vi "main.vi"() -> ()   [LabVIEW 2020]
uses:
  midi-ui/midi-ui.lvclass
  <vilib>/addons/_JKI Toolkits/State Machine/_JKI_lib_State_Machine.llb/Select State(s)_err__jki_lib_state_machine.vi
  midi-file/midi-file.lvclass
  midi/midi.lvclass
  midiPlayer/midiPlayer.lvclass
  midi-file-events/midi-file-events.lvclass
panel:
  out "File Name":string
  in  "Connect":bool
  in  "Midi Device":u32 caption="Numeric"
  in  "File Open":bool
  in  "Stop":bool
  in  "Pause":bool
  in  "Play":bool
  out "Connected?":bool
  in  "Exit":bool
  out "picture":picture
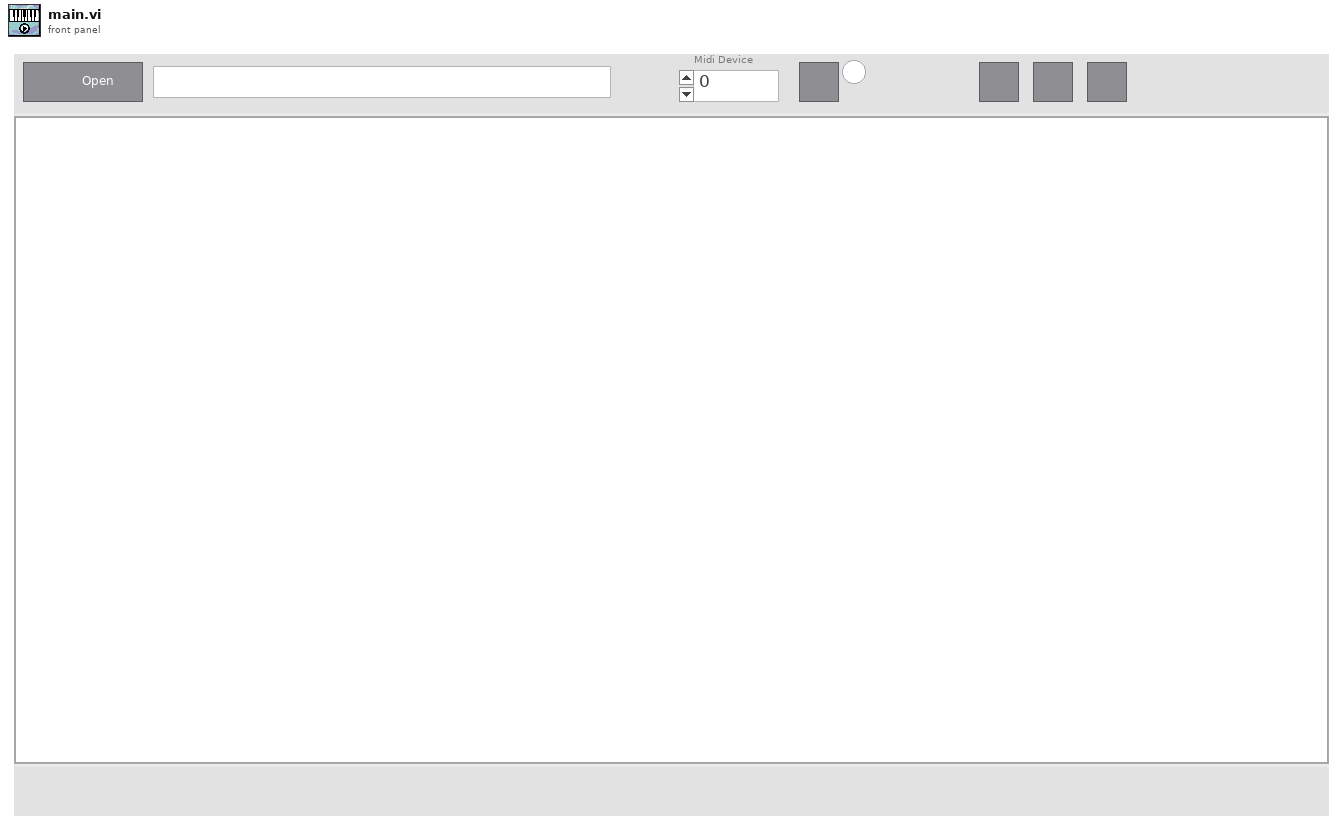
[diagram p1: front panel]
types:
  T1 = enum32{"Invalid", "Standard", "Closed", "Hidden", "Minimized", "Maximized"}
  T2 = enum32{"invalid app kind", "Development System", "Run Time System", "Student Edition", "Embedded LabVIEW", "Evaluation", "Custom"}
  T3 = cluster{"Core":cluster{"Current VI Reference":refnum<vi>, "Close Panel on Exit?":bool}, "MIDI UI":refnum<class "midi-ui.lvclass">, "midi-file-events":refnum<class "midi-file-events.lvclass">, "MIDI FILE":refnum<class "midi-file.lvclass">, "MIDI":refnum<class "midi.lvclass">, "midi connected?":bool, "midiPlayer":refnum<class "midiPlayer.lvclass">}
  T4 = cluster{"Current VI Reference":refnum<vi>, "Close Panel on Exit?":bool}
  T5 = typedef "configuration.ctl" = cluster{"Position":enum16{"Top", "Left", "Botom", "Right"}, "Note Length":dbl}
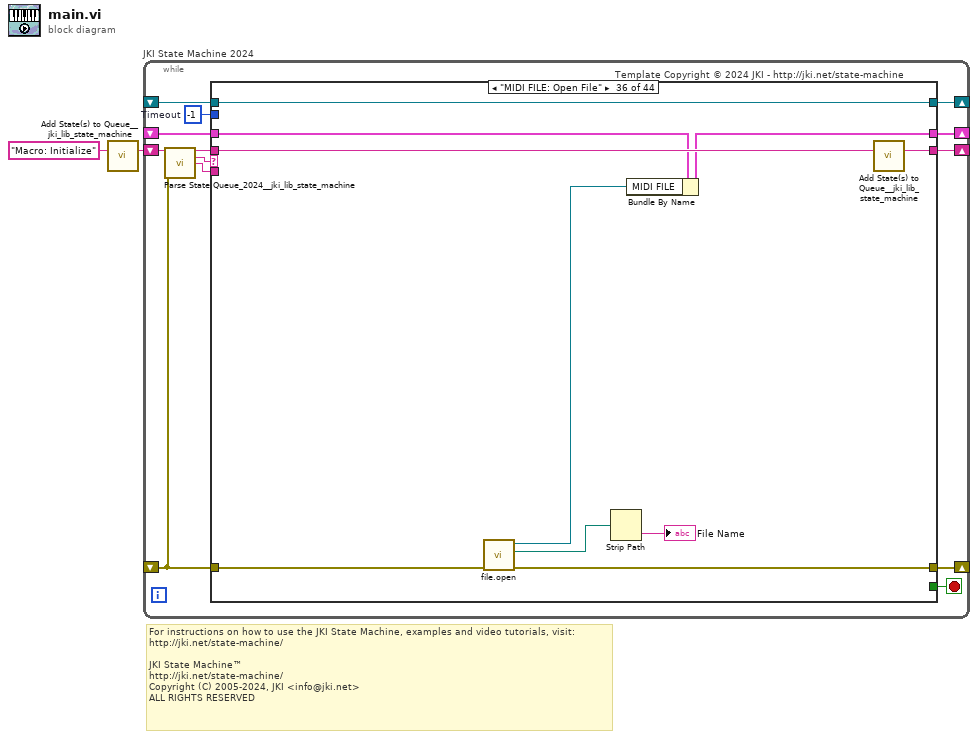
[diagram p0: block diagram]
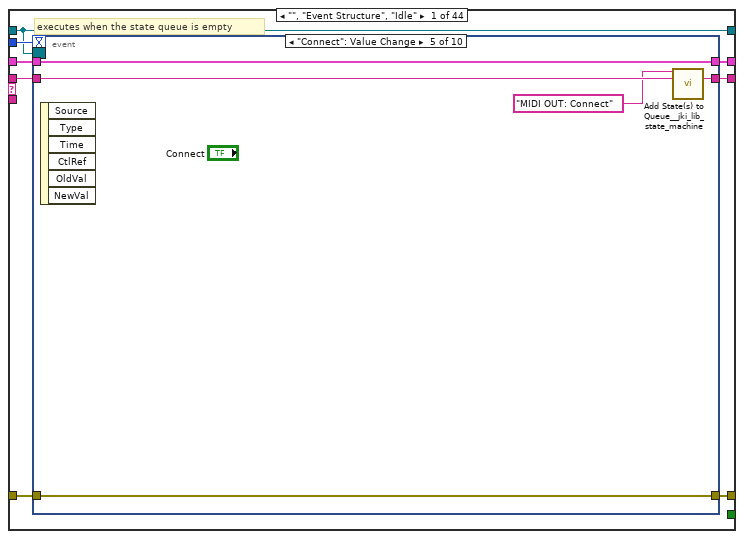
[diagram p2: hidden frame]
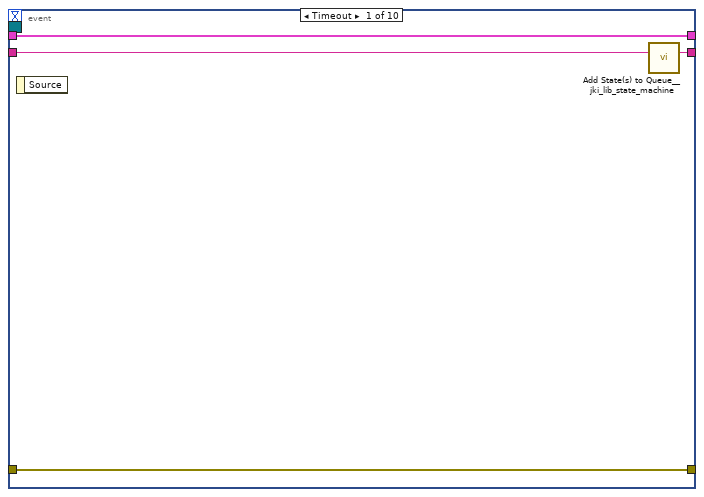
[diagram p3: hidden frame]
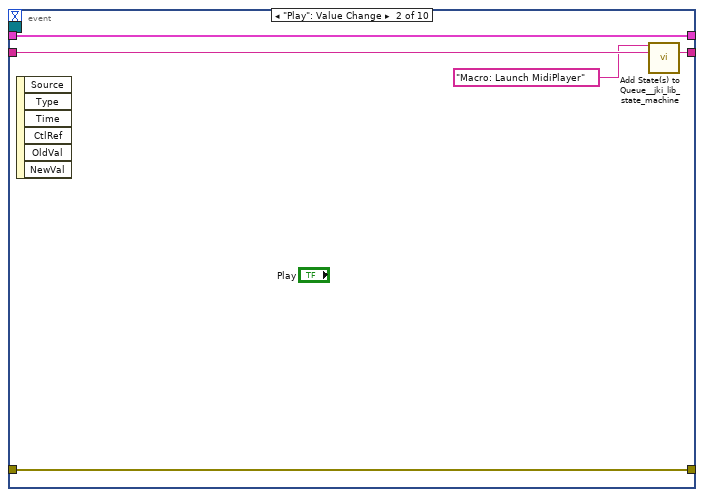
[diagram p4: hidden frame]
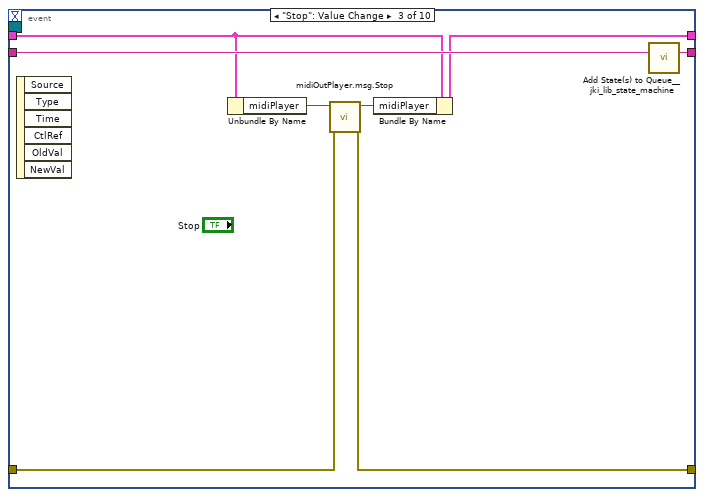
[diagram p5: hidden frame]
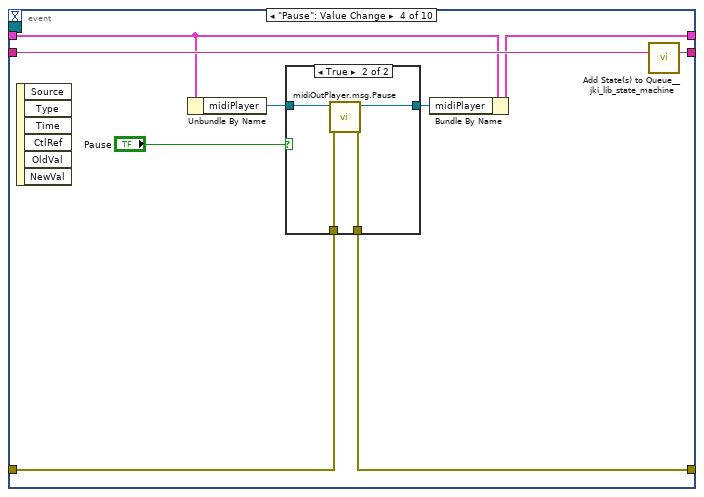
[diagram p6: hidden frame]
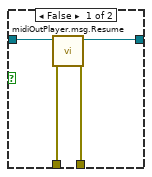
[diagram p7: hidden frame]
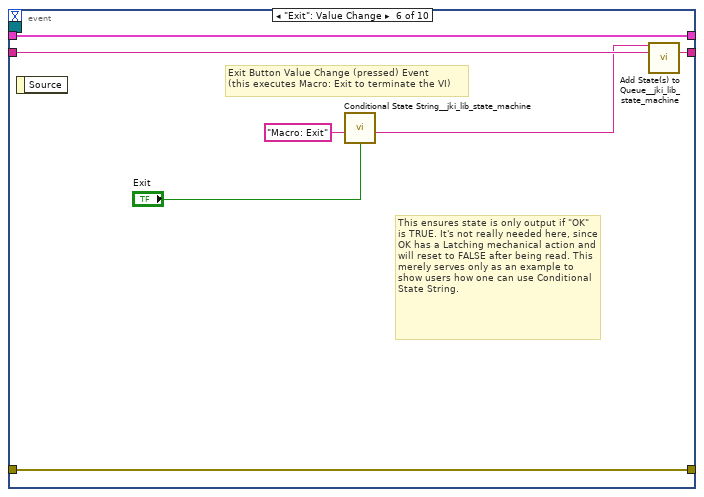
[diagram p8: hidden frame]
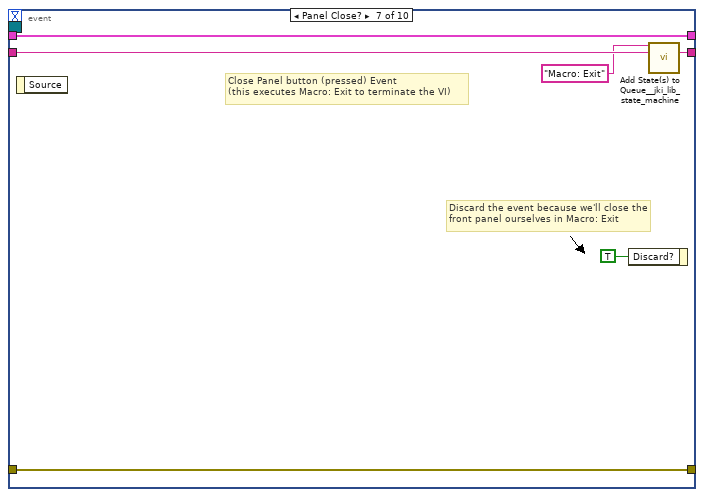
[diagram p9: hidden frame]
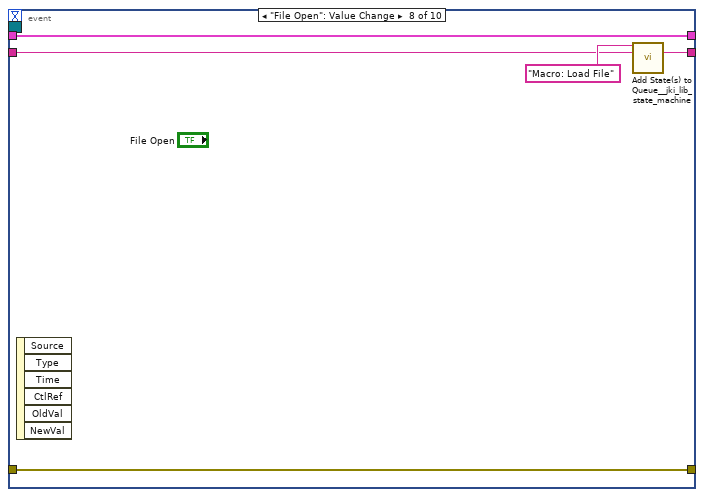
[diagram p10: hidden frame]
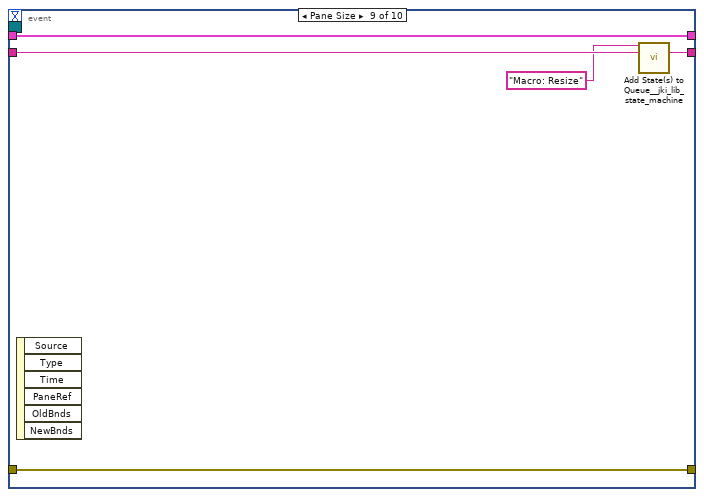
[diagram p11: hidden frame]
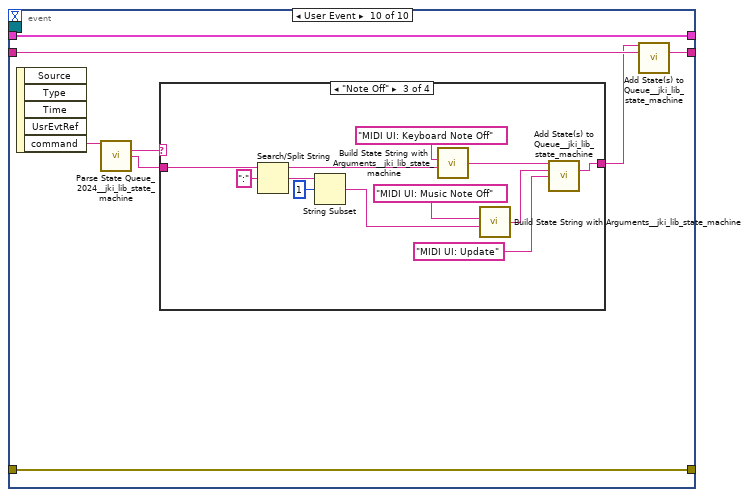
[diagram p12: hidden frame]
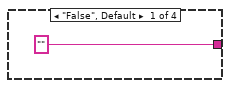
[diagram p13: hidden frame]
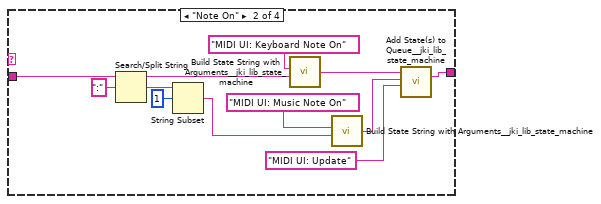
[diagram p14: hidden frame]
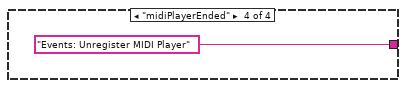
[diagram p15: hidden frame]
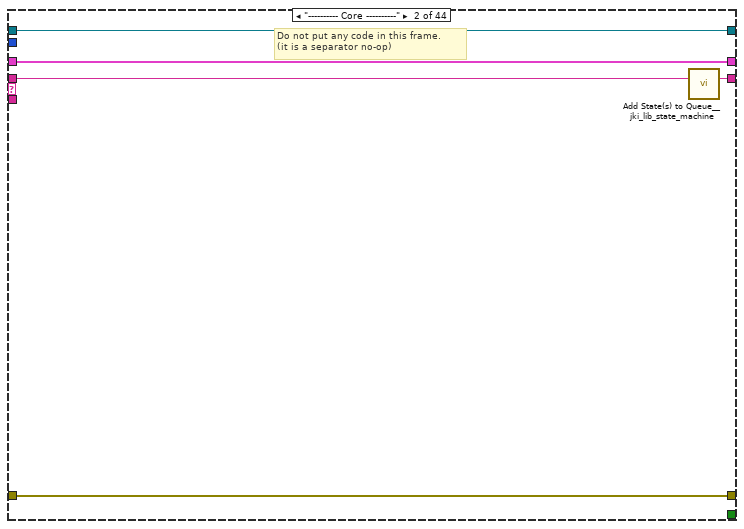
[diagram p16: hidden frame]
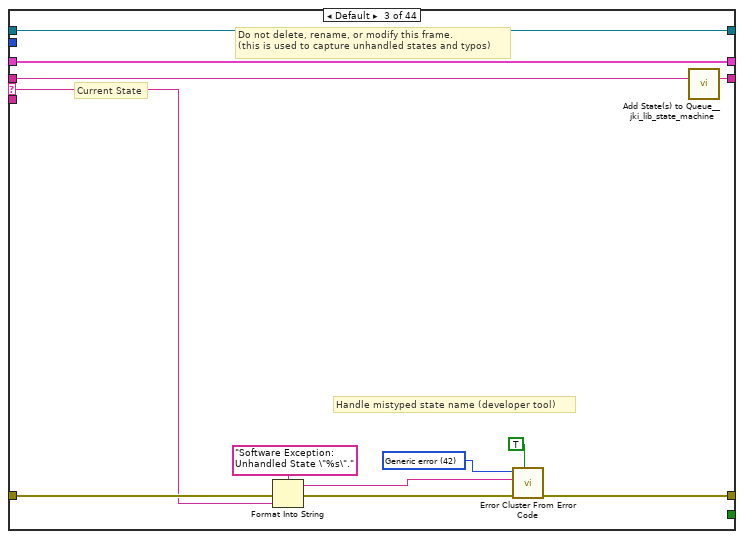
[diagram p17: hidden frame]
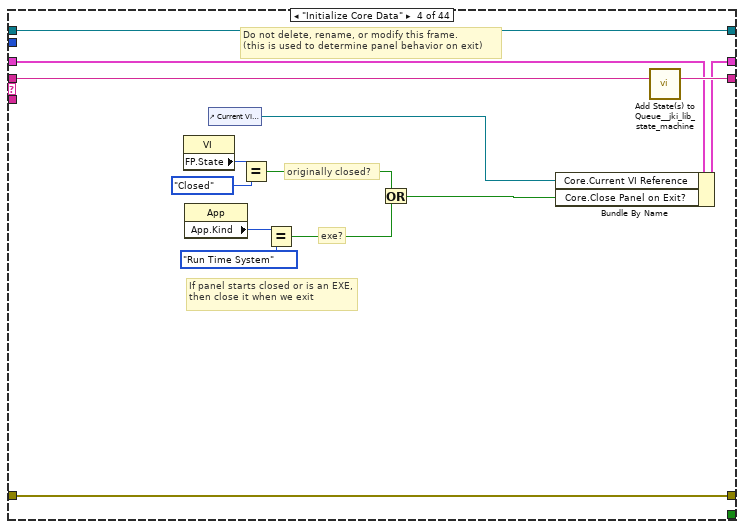
[diagram p18: hidden frame]
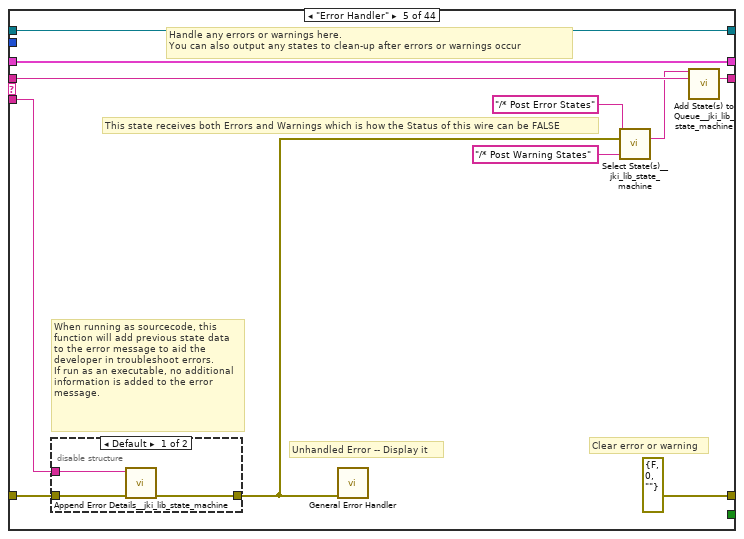
[diagram p19: hidden frame]
diagram:
  # "For instructions on how to use the JKI State Machine, examples and video tutorials, visit:\nhttp://jki.net/state-machine/\n\nJKI State Machine™\nhttp://jki.net/state-machine/\nCopyright (C) 2005-2024, JKI <info@jki.net>\nALL RIGHTS RESERVED"
  n1 = call <vilib>:"Add State(s) to Queue__jki_lib_state_machine.vi"("State(s) in (\"\")"="Macro: Initialize") -> ("States Out"=w2:string)  [unwired: 14 in]
  n2 = while "JKI State Machine 2024" {
    shift-right: [w10] -> _
    shift-left: _ -> [w9]
    shift-right: [w13] -> _
    shift-left: _ -> [w7]
    shift-right: [w12] -> _
    shift-left: w2 -> [w14]
    shift-right: [w4] -> _
    shift-left: _ -> [w3]
    stop <- w11 stop-if-true
    w8 = -1  # Timeout
    # "Template Copyright © 2024 JKI - http://jki.net/state-machine"
    n3 = call <vilib>:"Parse State Queue_2024__jki_lib_state_machine.vi"("State Queue"=w14, "Error In (no error)"=w7) -> ("Remaining States"=w15:string, "Current State"=w5:string, "Arguments"=w6:string)  [unwired: 11 in]
    n4 = case shown="\"MIDI FILE: Open File\"" w5 {
      selector: w5 -> [_ _ w126 _ _ _ _ _ _ _ _ _ _ _ _ _ _ _ _ _ _ _ _ _ _ _ _ _ _ _ _ _ _ _ _ _ _ _ _ _ _ _ _ _]
      tunnel: w15 -> [w23 w124 w130 w150 w161 w171 w176 w193 w204 w209 w216 w225 w233 w239 w244 w250 w255 w262 w274 w344 w350 w356 w362 w368 w381 w386 w395 w411 w421 w433 w441 w460 w476 w495 w506 w517 w528 w535 w540 w551 w561 w566 w580 w589]
      tunnel: w6 -> [_ _ _ _ w156 _ _ _ _ _ _ _ _ _ _ _ _ w257 w268 _ _ _ _ _ _ _ _ _ _ _ w434 w453 w469 w490 _ _ _ _ _ _ _ _ _ _]
      tunnel: w9 -> [w21 w121 w128 w143 w158 w169 w173 _ w200 w206 w214 w220 w231 w237 w241 w248 w253 w260 w270 w341 w347 w353 w359 w365 w379 w383 w388 w409 w418 w425 w439 w458 w474 w493 w508 w515 w526 w534 w539 w547 w557 w563 w577 w587]
      tunnel: [w20 w122 w132 w147 errorcluster {"status"=FALSE, "code"=0, "source"=""} ("error out") w168 w174 w185 w194 w207 w213 w223 w230 w234 w242 w247 w252 w258 w271 w342 w348 w354 w360 w366 w376 w384 w391 w406 w413 w427 w435 w454 w470 w488 w505 w513 w523 w531 w538 w544 w555 w564 w578 w585] -> w13
      tunnel: w7 -> [w17 w122 w131 w147 w157 w168 w174 w188 w201 w207 w212 w222 w229 w235 w242 w247 w252 w259 w272 w342 w348 w354 w360 w366 w376 w384 w390 w397 w414 w428 w436 w455 w471 w489 w505 w516 w524 w532 w538 w550 w556 w564 w568 w586]
      tunnel: [w22 w123 w129 w149 w160 w170 w175 w192 w203 w208 w215 w224 w232 w238 w243 w249 w254 w261 w273 w343 w349 w355 w361 w367 w380 w385 w394 w410 w420 w432 w440 w459 w475 w494 w507 w518 w529 w536 w541 w552 w562 w567 w581 w590] -> w12
      tunnel: [_ _ _ _ _ TRUE _ _ _ _ _ _ _ _ _ _ _ _ _ _ _ _ _ _ _ _ _ _ _ _ _ _ _ _ _ _ _ _ _ _ _ _ _ _] -> w11
      tunnel: [w19 w121 w128 w148 w158 w169 w173 w191 w200 w206 w214 w220 w231 w237 w241 w248 w253 w260 w270 w341 w347 w353 w359 w365 w379 w383 w389 w408 w419 w424 w438 w457 w473 w492 w508 w514 w527 w534 w539 w548 w560 w563 w576 w584] -> w10
      tunnel: w8 -> [w18 _ _ _ _ _ _ _ _ _ _ _ _ _ _ _ _ _ _ _ _ _ _ _ _ _ _ _ _ _ _ _ _ _ _ _ _ _ _ _ _ _ _ _]
      tunnel: [w16 w120 w125 w137 w151 w166 w172 w180 w199 w205 w210 w219 w226 w236 w240 w246 w251 w256 w267 w340 w346 w351 w357 w363 w373 w382 w393 w405 w417 w422 w437 w456 w472 w491 w504 w511 w521 w530 w537 w545 w554 w565 w579 w588] -> w4
      tunnel: w3 -> [w16 w120 w125 w137 w151 w166 w172 w180 w199 w205 w211 w218 w228 w236 w240 w246 w251 w256 w267 w340 w346 w351 w357 w363 w373 w382 w393 w405 w417 w422 w437 w456 w472 w491 w504 w511 w521 w530 w537 w545 w554 w565 w579 w588]
      frame "", "Event Structure", "Idle" {
        # "executes when the state queue is empty"
        n5 = event shown="[4] \"Connect\": Value Change" {
          selector: w16 -> [_ _ _ _ _ _ _ _ _ _]
          dyn-events: _ -> [_ _ _ _ _ _ _ _ _ _]
          timeout: w18 -> [_ _ _ _ _ _ _ _ _ _]
          tunnel: w23 -> [w27 w32 w40 w49 w62 w69 w75 w79 w83 w91]
          tunnel: [w26 w31 w39 w48 w61 w68 w74 w78 w84 w92] -> w22
          tunnel: w21 -> [w24 w29 w38 w46 w59 w66 w72 w77 w85 w86]
          tunnel: [w25 w30 w35 w43 w60 w67 w73 w76 w82 w93] -> w20
          tunnel: w17 -> [w25 w30 w36 w44 w60 w67 w73 w76 w82 w93]
          tunnel: [w24 w29 w37 w45 w59 w66 w72 w77 w85 w86] -> w19
          event Timeout {
            n6 = event-data() -> ()  [unwired: 1 in, 1 out]
            n7 = call <vilib>:"Add State(s) to Queue__jki_lib_state_machine.vi"("State(s) in (\"\")"=w27) -> ("States Out"=w26:string)  [unwired: 14 in]
          }
          event "Play": Value Change {
            n8 = event-data() -> ()  [unwired: 1 in, 6 out]
            n9 = call <vilib>:"Add State(s) to Queue__jki_lib_state_machine.vi"("State(s) in Front (\"\")"="Macro: Launch MidiPlayer" ("State(s) in Front (\"\")"), "State(s) in (\"\")"=w32) -> ("States Out"=w31:string)  [unwired: 13 in]
          }
          event "Stop": Value Change {
            n10 = event-data() -> ()  [unwired: 1 in, 6 out]
            n11 = Unbundle By Name(w38) -> ("midiPlayer"=w34:refnum<class "midiPlayer.lvclass">)
            n12 = call "midiOutPlayer.msg.Stop.vi"("error in (no error)"=w36, "midiPlayer in"=w34) -> ("error out"=w35:errorcluster, "midiPlayer out"=w33:refnum<class "midiPlayer.lvclass">)  [unwired: 8 in]
            n13 = Bundle By Name(cluster=w38, "midiPlayer"=w33) -> (w37:T3)
            n14 = call <vilib>:"Add State(s) to Queue__jki_lib_state_machine.vi"("State(s) in (\"\")"=w40) -> ("States Out"=w39:string)  [unwired: 14 in]
          }
          event "Pause": Value Change {
            n15 = event-data() -> ()  [unwired: 1 in, 6 out]
            n16 = Unbundle By Name(w46) -> ("midiPlayer"=w47:refnum<class "midiPlayer.lvclass">)
            n17 = case shown="True" "Pause" {
              tunnel: w47 -> [w50 w54]
              tunnel: [w52 w57] -> w42
              tunnel: w44 -> [w53 w56]
              tunnel: [w51 w55] -> w43
              frame False {
                n18 = call "midiOutPlayer.msg.Resume.vi"("error in (no error)"=w53, "midiPlayer in"=w50) -> ("error out"=w51:errorcluster, "midiPlayer out"=w52:refnum<class "midiPlayer.lvclass">)  [unwired: 8 in]
              }
              frame True {
                n19 = call "midiOutPlayer.msg.Pause.vi"("error in (no error)"=w56, "midiPlayer in"=w54) -> ("error out"=w55:errorcluster, "midiPlayer out"=w57:refnum<class "midiPlayer.lvclass">)  [unwired: 8 in]
              }
            }
            n20 = Bundle By Name(cluster=w46, "midiPlayer"=w42) -> (w45:T3)
            n21 = call <vilib>:"Add State(s) to Queue__jki_lib_state_machine.vi"("State(s) in (\"\")"=w49) -> ("States Out"=w48:string)  [unwired: 14 in]
          }
          event "Connect": Value Change {
            n22 = event-data() -> ()  [unwired: 1 in, 6 out]
            n23 = call <vilib>:"Add State(s) to Queue__jki_lib_state_machine.vi"("State(s) in Front (\"\")"="MIDI OUT: Connect" ("State(s) in Front (\"\")"), "State(s) in (\"\")"=w62) -> ("States Out"=w61:string)  [unwired: 13 in]
          }
          event "Exit": Value Change {
            # "This ensures state is only output if \"OK\" is TRUE. It's not really needed here, since OK has a Latching mechanical action and will reset to FALSE after being read. This merely serves only as an example to show users how one can use Conditional State String."
            # "Exit Button Value Change (pressed) Event\n(this executes Macro: Exit to terminate the VI)"
            n24 = event-data() -> ()  [unwired: 1 in, 1 out]
            n25 = call <vilib>:"Conditional State String__jki_lib_state_machine.vi"("Do State(s)?"="Exit", "State"="Macro: Exit") -> ("State Out"=w63:string)  [unwired: 7 in]
            n26 = call <vilib>:"Add State(s) to Queue__jki_lib_state_machine.vi"("State(s) in Front (\"\")"=w63, "State(s) in (\"\")"=w69) -> ("States Out"=w68:string)  [unwired: 13 in]
          }
          event Panel Close? {
            # "Discard the event because we'll close the front panel ourselves in Macro: Exit"
            # "Close Panel button (pressed) Event\n(this executes Macro: Exit to terminate the VI)"
            n27 = event-data() -> ()  [unwired: 1 in, 1 out]
            n28 = event-data("Discard?"=TRUE) -> ()  [unwired: 1 in, 1 out]
            n29 = call <vilib>:"Add State(s) to Queue__jki_lib_state_machine.vi"("State(s) in Front (\"\")"="Macro: Exit", "State(s) in (\"\")"=w75) -> ("States Out"=w74:string)  [unwired: 13 in]
          }
          event "File Open": Value Change {
            n30 = event-data() -> ()  [unwired: 1 in, 6 out]
            n31 = call <vilib>:"Add State(s) to Queue__jki_lib_state_machine.vi"("State(s) in Front (\"\")"="Macro: Load File", "State(s) in (\"\")"=w79) -> ("States Out"=w78:string)  [unwired: 13 in]
          }
          event Pane Size {
            n32 = event-data() -> ()  [unwired: 1 in, 6 out]
            n33 = call <vilib>:"Add State(s) to Queue__jki_lib_state_machine.vi"("State(s) in Front (\"\")"="Macro: Resize" ("State(s) in Front (\"\")"), "State(s) in (\"\")"=w83) -> ("States Out"=w84:string)  [unwired: 13 in]
          }
          event User Event {
            n34 = event-data() -> ("command"=w90:string)  [unwired: 1 in, 4 out]
            n35 = call <vilib>:"Parse State Queue_2024__jki_lib_state_machine.vi"("State Queue"=w90) -> ("Current State"=w89:string, "Arguments"=w87:string)  [unwired: 12 in, 1 out]
            n36 = case shown="\"Note Off\"" w89 {
              tunnel: ["" ("State(s) in Front (\"\")") w96 w118 "Events: Unregister MIDI Player" ("State(s) in Front (\"\")")] -> w88
              tunnel: w87 -> [_ w95 w107 _]
              frame "False", Default {
              }
              frame "Note On" {
                n37 = Search/Split String(string=w95, search string/char (-)=":") -> (substring before match=w103:string, match + rest of string=w102:string)  [unwired: 1 in, 1 out]
                n38 = String Subset(string=w102, offset (0)=1) -> (substring=w98:string)  [unwired: 1 in]
                n39 = call <vilib>:"Build State String with Arguments__jki_lib_state_machine.vi"("Arguments (\"\")"=w103, "State"="MIDI UI: Keyboard Note On" ("State(s) in Front (\"\")")) -> ("State with Arguments"=w105:string)  [unwired: 4 in]
                n40 = call <vilib>:"Build State String with Arguments__jki_lib_state_machine.vi"("Arguments (\"\")"=w98, "State"="MIDI UI: Music Note On" ("State(s) in Front (\"\")")) -> ("State with Arguments"=w97:string)  [unwired: 4 in]
                n41 = call <vilib>:"Add State(s) to Queue__jki_lib_state_machine.vi"("State(s) in Front (\"\")"=w105, "State(s) in (\"\")"=w97, "State(s) at Back (\"\")"="MIDI UI: Update" ("State(s) in (\"\")")) -> ("States Out"=w96:string)  [unwired: 12 in]
              }
              frame "Note Off" {
                n42 = Search/Split String(string=w107, search string/char (-)=":") -> (substring before match=w114:string, match + rest of string=w113:string)  [unwired: 1 in, 1 out]
                n43 = String Subset(string=w113, offset (0)=1) -> (substring=w109:string)  [unwired: 1 in]
                n44 = call <vilib>:"Build State String with Arguments__jki_lib_state_machine.vi"("Arguments (\"\")"=w114, "State"="MIDI UI: Keyboard Note Off" ("State(s) in Front (\"\")")) -> ("State with Arguments"=w116:string)  [unwired: 4 in]
                n45 = call <vilib>:"Build State String with Arguments__jki_lib_state_machine.vi"("Arguments (\"\")"=w109, "State"="MIDI UI: Music Note Off" ("State(s) in Front (\"\")")) -> ("State with Arguments"=w108:string)  [unwired: 4 in]
                n46 = call <vilib>:"Add State(s) to Queue__jki_lib_state_machine.vi"("State(s) in Front (\"\")"=w116, "State(s) in (\"\")"=w108, "State(s) at Back (\"\")"="MIDI UI: Update" ("State(s) in (\"\")")) -> ("States Out"=w118:string)  [unwired: 12 in]
              }
              frame "midiPlayerEnded" {
              }
            }
            n47 = call <vilib>:"Add State(s) to Queue__jki_lib_state_machine.vi"("State(s) in Front (\"\")"=w88, "State(s) in (\"\")"=w91) -> ("States Out"=w92:string)  [unwired: 13 in]
          }
        }
      }
      frame "---------- Core ----------" {
        # "Do not put any code in this frame.\n(it is a separator no-op)"
        n48 = call <vilib>:"Add State(s) to Queue__jki_lib_state_machine.vi"("State(s) in (\"\")"=w124) -> ("States Out"=w123:string)  [unwired: 14 in]
      }
      frame Default {
        w135 = 42 items=["No error", "Argument error", "Memory is full", "Out of zone", "End of file", "File already open", "Generic file I/O error", "File not found", "File permission error", "Disk is full", "Duplicate path", "Too many files open", "System feature not enabled", "Resource file not found", "Cannot add resource", "Resource not found", "Image not found", "Image memory error", "Pen does not exist", "Config type invalid", "Config token not found", "Config parse error", "Config memory error", "Bad external code format", "Bad external code offset", "External code not present", "Null window", "Destroy window error", "Null menu", "Print aborted", "Bad print record", "Print driver error", "Windows error during printing", "Memory error during printing", "Print dialog error", "Generic print error", "Invalid device refnum", "Device not found", "Device parameter error", "Device unit error", "Cannot open device", "Device call aborted", "Generic error", "Cancelled by user", "Object ID too low", "Object ID too high", "Object not in heap", "Unknown heap", "Unknown object (invalid DefProc)", "Unknown object (DefProc not in table)", "Message out of range", "Invalid (null) method", "Unknown message", "Manager call not supported", "Bad address", "Network operation in progress", "Network operation timed out", "Connection is busy", "Network attribute not supported", "Network error", "Address in use", "System out of memory", "Connection aborted", "Connection refused", "Not connected", "Already connected", "Connection closed", "Initialization error (interapplication manager)", "Bad occurrence", "Wait on unbound occurrence handler", "Occurrence queue overflow", "Datalog type conflict", "Unused", "Unrecognized type (interapplication manager)", "Memory corrupt", "Failed to make temporary DLL", "Old CIN version", "Drag socket not found", "Failed to load drop-object", "Failed to register OLE object", "Failed to release OLE object", "Format specifier type mismatch", "Unknown format specifier", "Too few format specifiers", "Too many format specifiers", "Scan failed", "Newer CIN version", "Error converting to variant", "Runtime menu error", "Password tampered", "Variant attribute not found", "Incompatible variant data type", "Event data is not available", "Event Store is not present", "Occurrence is not found", "Event Queue is not created", "Event info is not available", "Refnum passed is NULL", "Error retrieving Class GUID", "Error retrieving CoClass GUID", "Error retrieving TypeLib GUID.", "Bad built application magic bytes.", "Specific driver is different from the specific driver associated with the Logical Name.", "There is no session opened to the class driver.", "Max Error", "MAX - Error with config objects", "MAX - Error loading configuration", "MAX - Group not supported"]
        # "Current State"
        # "Do not delete, rename, or modify this frame.\n(this is used to capture unhandled states and typos)"
        # "Handle mistyped state name (developer tool)"
        n49 = Format Into String(format string="Software Exception: Unhandled State \"%s\"." ("message"), error in=w131, w126) -> (resulting string=w134:string, error out=w133:errorcluster)  [unwired: 1 in]
        n50 = call <vilib>:"Error Cluster From Error Code.vi"("show call chain? (False)"=TRUE, "error in (no error)"=w133, "error message (\"\")"=w134, "error code (0)"=w135) -> ("error out"=w132:errorcluster)  [unwired: 5 in]
        n51 = call <vilib>:"Add State(s) to Queue__jki_lib_state_machine.vi"("State(s) in (\"\")"=w130) -> ("States Out"=w129:string)  [unwired: 14 in]
      }
      frame "Initialize Core Data" {
        # "Do not delete, rename, or modify this frame.\n(this is used to determine panel behavior on exit)"
        # "originally closed?"
        # "exe?"
        # "If panel starts closed or is an EXE, then close it when we exit"
        n52 = property class="VI"() -> ("FP.State"=w140:T1)  [unwired: 2 in, 2 out]
        n53 = property class="App"() -> ("App.Kind"=w146:T2)  [unwired: 2 in, 2 out]
        n54 = control-ref of="Current VI Reference"() -> (w141:refnum<vi>)
        n55 = Equal?(x=w140, y=T1."Closed" ("Front Panel Window:State")) -> (x = y?=w138:bool)
        n56 = Equal?(x=w146, y=T2."Run Time System" ("Application:Kind")) -> (x = y?=w144:bool)
        n57 = Or(x=w138, y=w144) -> (x .or. y?=w142:bool)
        n58 = Bundle By Name(cluster=w143, "Core.Current VI Reference"=w141, "Core.Close Panel on Exit?"=w142) -> (w148:T3)
        n59 = call <vilib>:"Add State(s) to Queue__jki_lib_state_machine.vi"("State(s) in (\"\")"=w150) -> ("States Out"=w149:string)  [unwired: 14 in]
      }
      frame "Error Handler" {
        # "When running as sourcecode, this function will add previous state data to the error message to aid the developer in troubleshoot errors.\nIf run as an executable, no additional information is added to the error message."
        # "This state receives both Errors and Warnings which is how the Status of this wire can be FALSE"
        # "Unhandled Error -- Display it"
        # "Handle any errors or warnings here.\nYou can also output any states to clean-up after errors or warnings occur"
        # "Clear error or warning"
        n60 = disable-structure shown="Default" {
          disable-tunnel: w157 -> [w164 w165]
          disable-tunnel: w156 -> [w163 _]
          disable-tunnel: [w162 w165] -> w155
          frame condition #0 (active) {
            n61 = call <vilib>:"Append Error Details__jki_lib_state_machine.vi"("error in (no error)"=w164, "Previous State and Argument(s)"=w163) -> ("error out"=w162:errorcluster)  [unwired: 9 in]
          }
          frame condition #1 {
          }
        }
        n62 = call <vilib>:"General Error Handler.vi"("error in (no error)"=w155) -> ()  [unwired: 10 in, 5 out]
        n63 = call-poly <vilib>:"Select State(s)__jki_lib_state_machine.vi"("State(s) if True (\"\")"="/* Post Error States", "Select"=w155, "State(s) if False (\"\")"="/* Post Warning States") -> ("States Out"=w153:string)  [unwired: 12 in]
        n64 = call <vilib>:"Add State(s) to Queue__jki_lib_state_machine.vi"("State(s) in Front (\"\")"=w153, "State(s) in (\"\")"=w161) -> ("States Out"=w160:string)  [unwired: 13 in]
      }
      frame "Exit" {
        # "Do not put any code in this frame.\n(No errors that occur here will be handled.)"
        n65 = call <vilib>:"Add State(s) to Queue__jki_lib_state_machine.vi"("State(s) in (\"\")"=w171) -> ("States Out"=w170:string)  [unwired: 14 in]
      }
      frame "---------- Data ----------" {
        # "Do not put any code in this frame.\n(It is a separator no-op. You can make a copy of this frame to create a new Data frame)"
        n66 = call <vilib>:"Add State(s) to Queue__jki_lib_state_machine.vi"("State(s) in (\"\")"=w176) -> ("States Out"=w175:string)  [unwired: 14 in]
      }
      frame "Data: Initialize" {
        w178 = refnum<class "midiPlayer.lvclass"> refnum  # midiPlayer
        w179 = FALSE  # midi connected?
        w181 = refnum<class "midi.lvclass"> refnum  # MIDI
        w184 = refnum<class "midi-file.lvclass"> refnum  # MIDI FILE
        w186 = refnum<class "midi-ui.lvclass"> refnum  # MIDI UI
        w190 = T4 {"Current VI Reference"=refnum, "Close Panel on Exit?"=FALSE}  # Core
        # "Data names and types of shift register data are defined by this bundle."
        # "Initialize the shift-register data, here.\n(data names are defined by what you wire into the bundle function)"
        n67 = control-ref of="picture"() -> (w189:refnum<vi>)
        n68 = call "create.vi"("Picture Control"=w189, "error in (no error)"=w188) -> ("error out"=w182:errorcluster, "midi-ui out"=w183:refnum<class "midi-ui.lvclass">)  [unwired: 8 in]
        n69 = Variant To Data(error in=w182, type=w186, Variant=w183) -> (data=w187:refnum<class "midi-ui.lvclass">, error out=w185:errorcluster)
        n70 = call "create.vi"() -> ("midi-file-events"=w177:refnum<class "midi-file-events.lvclass">)  [unwired: 10 in, 1 out]
        n71 = Bundle("Core"=w190, "MIDI UI"=w187, "midi-file-events"=w177, "MIDI FILE"=w184, "MIDI"=w181, "midi connected?"=w179, "midiPlayer"=w178) -> (w191:T3)  [unwired: 1 in]
        n72 = call <vilib>:"Add State(s) to Queue__jki_lib_state_machine.vi"("State(s) in (\"\")"=w193) -> ("States Out"=w192:string)  [unwired: 14 in]
      }
      frame "Data: Cleanup" {
        # "Cleanup any data and references, here.\n(this is called automatically, by the Macro: Exit)"
        n73 = Unbundle By Name(w200) -> ("midi-file-events"=w196:refnum<class "midi-file-events.lvclass">, "MIDI UI"=w198:refnum<class "midi-ui.lvclass">, "Core.Current VI Reference"=w202:refnum<vi>)
        n74 = Close Reference(reference=w202, error in (no error)=w201) -> (error out=w197:errorcluster)
        n75 = call "close.vi"("error in (no error)"=w197, "midi-ui in"=w198) -> ("error out"=w195:errorcluster)  [unwired: 9 in]
        n76 = call "destroy.vi"("error in (no error)"=w195, "midi-file-events"=w196) -> ("error out"=w194:errorcluster)  [unwired: 9 in]
        n77 = call <vilib>:"Add State(s) to Queue__jki_lib_state_machine.vi"("State(s) in (\"\")"=w204) -> ("States Out"=w203:string)  [unwired: 14 in]
      }
      frame "---------- Events ----------" {
        # "Do not put any code in this frame.\n(It is a separator no-op. You can make a copy of this frame to create a new UI frame)"
        n78 = call <vilib>:"Add State(s) to Queue__jki_lib_state_machine.vi"("State(s) in (\"\")"=w209) -> ("States Out"=w208:string)  [unwired: 14 in]
      }
      frame "Events: Register" {
        # "Do not put any code in this frame.\n(It is a separator no-op. You can make a copy of this frame to create a new UI frame)"
        n79 = register-events(reference=w211, error in=w212) -> (reference out=w210:refnum<event-registration>, error out=w213:errorcluster)  [unwired: 2 in]
        n80 = call <vilib>:"Add State(s) to Queue__jki_lib_state_machine.vi"("State(s) in (\"\")"=w216) -> ("States Out"=w215:string)  [unwired: 14 in]
      }
      frame "Events: Register MIDI Player" {
        # "Do not put any code in this frame.\n(It is a separator no-op. You can make a copy of this frame to create a new UI frame)"
        n81 = Unbundle By Name(w220) -> ("midiPlayer"=w217:refnum<class "midiPlayer.lvclass">)
        n82 = call "midiPlayer.announcements.get.vi"("midiPlayer"=w217) -> ("midiPlayer.Announcements"=w221:refnum<user-event>)  [unwired: 10 in]
        n83 = register-events(reference=w218, error in=w222, w221) -> (reference out=w219:refnum<event-registration>, error out=w223:errorcluster)  [unwired: 1 in]
        n84 = call <vilib>:"Add State(s) to Queue__jki_lib_state_machine.vi"("State(s) in (\"\")"=w225) -> ("States Out"=w224:string)  [unwired: 14 in]
      }
      frame "Events: Unregister MIDI Player" {
        # "Do not put any code in this frame.\n(It is a separator no-op. You can make a copy of this frame to create a new UI frame)"
        n85 = register-events(reference=w228, error in=w229, refnum<user-event> refnum ("event source")) -> (reference out=w226:refnum<event-registration>, error out=w230:errorcluster)  [unwired: 1 in]
        n86 = call <vilib>:"Add State(s) to Queue__jki_lib_state_machine.vi"("State(s) in (\"\")"=w233) -> ("States Out"=w232:string)  [unwired: 14 in]
      }
      frame "Events: Unregister" {
        # "Do not put any code in this frame.\n(It is a separator no-op. You can make a copy of this frame to create a new UI frame)"
        n87 = Unregister For Events(event registration refnum=w236, error in=w235) -> (error out=w234:errorcluster)
        n88 = call <vilib>:"Add State(s) to Queue__jki_lib_state_machine.vi"("State(s) in (\"\")"=w239) -> ("States Out"=w238:string)  [unwired: 14 in]
      }
      frame "---------- UI ----------" {
        # "Do not put any code in this frame.\n(It is a separator no-op. You can make a copy of this frame to create a new UI frame)"
        n89 = call <vilib>:"Add State(s) to Queue__jki_lib_state_machine.vi"("State(s) in (\"\")"=w244) -> ("States Out"=w243:string)  [unwired: 14 in]
      }
      frame "UI: Initialize" {
        # "Initialize the User Interface, here.\n(this is called automatically, by the Macro: Initialize)"
        n90 = local write "Pause"(FALSE ("Pause")) -> ()
        n91 = call <vilib>:"Add State(s) to Queue__jki_lib_state_machine.vi"("State(s) in (\"\")"=w250) -> ("States Out"=w249:string)  [unwired: 14 in]
      }
      frame "UI: Uninitialize" {
        # "Cleanup the User Interface, here.\n(this is called automatically, by the Macro: Exit)"
        n92 = call <vilib>:"Add State(s) to Queue__jki_lib_state_machine.vi"("State(s) in (\"\")"=w255) -> ("States Out"=w254:string)  [unwired: 14 in]
      }
      frame "UI: Cursor Set" {
        # "Argument"
        # "Set and Unset Cursor Busy.\n(Usage: \"UI: Cursor Set >> Busy|Idle\")"
        n93 = case shown="\"Idle\", Default" w257 {
          tunnel: w259 -> [w264 w266]
          tunnel: [w263 w265] -> w258
          frame "Idle", Default {
            n94 = call <vilib>:"Unset Busy.vi"("error in (no error)"=w264) -> ("error out"=w263:errorcluster)  [unwired: 10 in]
          }
          frame "Busy" {
            n95 = call <vilib>:"Set Busy.vi"("error in (no error)"=w266) -> ("error out"=w265:errorcluster)  [unwired: 9 in, 1 out]
          }
        }
        n96 = call <vilib>:"Add State(s) to Queue__jki_lib_state_machine.vi"("State(s) in (\"\")"=w262) -> ("States Out"=w261:string)  [unwired: 14 in]
      }
      frame "UI: Front Panel State" {
        # "Argument"
        # "Set Front Panel Open or Closed\n(Usage: \"UI: Front Panel State >> Open|Close\")"
        n97 = Unbundle By Name(w270) -> ("Core.Current VI Reference"=w269:refnum<vi>)
        n98 = case shown="\"Minimize\", \"Minimized\"" w268 {
          tunnel: w272 -> [w280 w295 w306 w319 w332]
          tunnel: [w282 w296 w308 w321 w334] -> w271
          tunnel: w269 -> [w281 w293 w307 w320 w333]
          frame "Open", "Standard", Default {
            w275 = T1."Standard" ("State")
            n99 = property class="VI"(reference=w281, error in=w280) -> (reference out=w278:refnum<vi>, error out=w279:errorcluster, "FP.State"=w277:T1)
            n100 = Not Equal?(x=w277, y=w275) -> (x != y?=w276:bool)
            n101 = case shown="True" w276 {
              tunnel: [w286 w288] -> w282
              tunnel: w279 -> [w285 w288]
              tunnel: w278 -> [w284 _]
              tunnel: w275 -> [w283 _]
              frame True {
                n102 = invoke class="VI" method="FP.Open"(reference=w284, error in=w285, "Activate"=TRUE, "State"=w283) -> (error out=w286:errorcluster)  [unwired: 1 in, 4 out]
              }
              frame False {
              }
            }
          }
          frame "Close", "Closed" {
            n103 = property class="VI"(reference=w293, error in=w295) -> (reference out=w292:refnum<vi>, error out=w294:errorcluster, "FP.State"=w290:T1)
            n104 = Not Equal?(x=w290, y=T1."Closed" ("Front Panel Window:State")) -> (x != y?=w289:bool)
            n105 = case shown="True" w289 {
              tunnel: [w297 w300] -> w296
              tunnel: w294 -> [w297 w299]
              tunnel: w292 -> [_ w298]
              frame False {
              }
              frame True {
                n106 = invoke class="VI" method="FP.Close"(reference=w298, error in=w299) -> (error out=w300:errorcluster)  [unwired: 1 in, 2 out]
              }
            }
          }
          frame "Hidden", "Hide" {
            w301 = T1."Hidden" ("State")
            n107 = property class="VI"(reference=w307, error in=w306) -> (reference out=w304:refnum<vi>, error out=w305:errorcluster, "FP.State"=w303:T1)
            n108 = Not Equal?(x=w303, y=w301) -> (x != y?=w302:bool)
            n109 = case shown="True" w302 {
              tunnel: [w312 w313] -> w308
              tunnel: w305 -> [w311 w313]
              tunnel: w304 -> [w310 _]
              tunnel: w301 -> [w309 _]
              frame True {
                n110 = invoke class="VI" method="FP.Open"(reference=w310, error in=w311, "State"=w309) -> (error out=w312:errorcluster)  [unwired: 2 in, 4 out]
              }
              frame False {
              }
            }
          }
          frame "Minimize", "Minimized" {
            w314 = T1."Minimized" ("State")
            n111 = property class="VI"(reference=w320, error in=w319) -> (reference out=w317:refnum<vi>, error out=w318:errorcluster, "FP.State"=w316:T1)
            n112 = Not Equal?(x=w316, y=w314) -> (x != y?=w315:bool)
            n113 = case shown="True" w315 {
              tunnel: [w325 w326] -> w321
              tunnel: w318 -> [w324 w326]
              tunnel: w317 -> [w323 _]
              tunnel: w314 -> [w322 _]
              frame True {
                n114 = invoke class="VI" method="FP.Open"(reference=w323, error in=w324, "State"=w322) -> (error out=w325:errorcluster)  [unwired: 2 in, 4 out]
              }
              frame False {
              }
            }
          }
          frame "Maximize", "Maximized" {
            w327 = T1."Maximized" ("State")
            n115 = property class="VI"(reference=w333, error in=w332) -> (reference out=w330:refnum<vi>, error out=w331:errorcluster, "FP.State"=w329:T1)
            n116 = Not Equal?(x=w329, y=w327) -> (x != y?=w328:bool)
            n117 = case shown="True" w328 {
              tunnel: [w338 w339] -> w334
              tunnel: w331 -> [w337 w339]
              tunnel: w330 -> [w336 _]
              tunnel: w327 -> [w335 _]
              frame True {
                n118 = invoke class="VI" method="FP.Open"(reference=w336, error in=w337, "State"=w335) -> (error out=w338:errorcluster)  [unwired: 2 in, 4 out]
              }
              frame False {
              }
            }
          }
        }
        n119 = call <vilib>:"Add State(s) to Queue__jki_lib_state_machine.vi"("State(s) in (\"\")"=w274) -> ("States Out"=w273:string)  [unwired: 14 in]
      }
      frame "---------- Macro ----------" {
        # "Do not put any code in this frame.\n(It is a separator no-op. You can make a copy of this frame to create a new Macro frame)"
        n120 = call <vilib>:"Add State(s) to Queue__jki_lib_state_machine.vi"("State(s) in (\"\")"=w344) -> ("States Out"=w343:string)  [unwired: 14 in]
      }
      frame "Macro: Launch MidiPlayer" {
        n121 = call <vilib>:"Add State(s) to Queue__jki_lib_state_machine.vi"("State(s) in Front (\"\")"="MIDI UI: Add Keyboard\nMIDI OUT: Launch Player\nEvents: Register MIDI Player\nMIDI OUT: Play" ("State(s) in Front (\"\")"), "State(s) in (\"\")"=w350) -> ("States Out"=w349:string)  [unwired: 13 in]
      }
      frame "Macro: Initialize" {
        # "Initialization Macro\n(This is called once, when the VI starts)"
        n122 = call <vilib>:"Add State(s) to Queue__jki_lib_state_machine.vi"("State(s) in Front (\"\")"="Data: Initialize\nInitialize Core Data\nEvents: Register\nUI: Initialize\nMIDI UI: Add Keyboard\nMIDI UI: Update\nUI: Front Panel State >> Open", "State(s) in (\"\")"=w356) -> ("States Out"=w355:string)  [unwired: 13 in]
      }
      frame "Macro: Load File" {
        n123 = call <vilib>:"Add State(s) to Queue__jki_lib_state_machine.vi"("State(s) in Front (\"\")"="MIDI FILE: Open File\nUI: Cursor Set >> Busy\nMIDI FILE: Analyse File\nMIDI FILE: Close File\nMIDI UI: Load File Data\nMIDI UI: Update\nUI: Cursor Set >> Idle" ("State(s) in Front (\"\")"), "State(s) in (\"\")"=w362) -> ("States Out"=w361:string)  [unwired: 13 in]
      }
      frame "Macro: Resize" {
        # "Do not put any code in this frame.\n(It is a separator no-op. You can make a copy of this frame to create a new Macro frame)"
        n124 = call <vilib>:"Add State(s) to Queue__jki_lib_state_machine.vi"("State(s) in Front (\"\")"="MIDI UI: Add Keyboard\nMIDI UI: Load File Data\nMIDI UI: Update" ("State(s) in Front (\"\")"), "State(s) in (\"\")"=w368) -> ("States Out"=w367:string)  [unwired: 13 in]
      }
      frame "Macro: Exit" {
        # "Exit Macro\n(This is called once, when the VI exits)"
        n125 = Unbundle By Name(w379) -> ("Core.Close Panel on Exit?"=w374:bool, "midi connected?"=w370:bool)
        n126 = call <vilib>:"Conditional State String__jki_lib_state_machine.vi"("Do State(s)?"=w370, "State"="MIDI OUT: Disconnect") -> ("State Out"=w369:string)  [unwired: 7 in]
        n127 = call <vilib>:"Conditional State String__jki_lib_state_machine.vi"("Do State(s)?"=w374, "State"="UI: Front Panel State >> Close") -> ("State Out"=w372:string)  [unwired: 7 in]
        n128 = call <vilib>:"Add State(s) to Queue__jki_lib_state_machine.vi"("State(s) in Front (\"\")"=w372, "State(s) in (\"\")"=w369, "State(s) at Back (\"\")"="MIDI UI: Clear Screen\nUI: Uninitialize\nData: Cleanup\nEvents: Unregister\nExit") -> ("States Out"=w377:string)  [unwired: 12 in]
        n129 = call <vilib>:"Add State(s) to Queue__jki_lib_state_machine.vi"("State(s) in Front (\"\")"=w377, "State(s) in (\"\")"=w381) -> ("States Out"=w380:string)  [unwired: 13 in]
      }
      frame "---------- MIDI UI ----------" {
        # "Template Separator\n(You can make a copy of, or modify, this frame)"
        n130 = call <vilib>:"Add State(s) to Queue__jki_lib_state_machine.vi"("State(s) in (\"\")"=w386) -> ("States Out"=w385:string)  [unwired: 14 in]
      }
      frame "MIDI UI: Update" {
        n131 = Unbundle By Name(w388) -> ("MIDI UI"=w392:refnum<class "midi-ui.lvclass">)
        n132 = call "picture.publish.vi"("error in"=w390, "midi-ui in"=w392) -> ("error out"=w391:errorcluster, "midi-ui out"=w387:refnum<class "midi-ui.lvclass">)  [unwired: 8 in]
        n133 = Bundle By Name(cluster=w388, "MIDI UI"=w387) -> (w389:T3)
        n134 = call <vilib>:"Add State(s) to Queue__jki_lib_state_machine.vi"("State(s) in (\"\")"=w395) -> ("States Out"=w394:string)  [unwired: 14 in]
      }
      frame "MIDI UI: Add Keyboard" {
        n135 = Unbundle By Name(w409) -> ("MIDI UI"=w400:refnum<class "midi-ui.lvclass">)
        n136 = call "picture.clear.vi"("Keep Keyboard? (T)"=FALSE, "error in"=w397, "midi-ui in"=w400) -> ("error out"=w398:errorcluster, "midi-ui out"=w399:refnum<class "midi-ui.lvclass">)  [unwired: 7 in]
        n137 = call "configuration.get.vi"("error in"=w398) -> ("error out"=w401:errorcluster, "configuration"=w404:T5)  [unwired: 9 in]
        n138 = Unbundle By Name(w404) -> ("Note Length"=w403:dbl, "Position"=w402:enum16{"Top", "Left", "Botom", "Right"})
        n139 = call "keyboard.add.vi"("Note Length (-1)"=w403, "error in (no error)"=w401, "Position"=w402, "midi-ui in"=w399) -> ("error out"=w406:errorcluster, "midi-ui out"=w407:refnum<class "midi-ui.lvclass">)  [unwired: 6 in]
        n140 = Bundle By Name(cluster=w409, "MIDI UI"=w407) -> (w408:T3)
        n141 = call <vilib>:"Add State(s) to Queue__jki_lib_state_machine.vi"("State(s) in (\"\")"=w411) -> ("States Out"=w410:string)  [unwired: 14 in]
      }
      frame "MIDI UI: Load File Data" {
        n142 = Unbundle By Name(w418) -> ("MIDI UI"=w416:refnum<class "midi-ui.lvclass">, "midi-file-events"=w415:refnum<class "midi-file-events.lvclass">)
        n143 = call "notes.add.vi"("error in (no error)"=w414, "midi-file-events"=w415, "midi-ui in"=w416) -> ("error out"=w413:errorcluster, "midi-ui out"=w412:refnum<class "midi-ui.lvclass">)  [unwired: 7 in]
        n144 = Bundle By Name(cluster=w418, "MIDI UI"=w412) -> (w419:T3)
        n145 = call <vilib>:"Add State(s) to Queue__jki_lib_state_machine.vi"("State(s) in (\"\")"=w421) -> ("States Out"=w420:string)  [unwired: 14 in]
      }
      frame "MIDI UI: Clear Screen" {
        n146 = Unbundle By Name(w425) -> ("MIDI UI"=w426:refnum<class "midi-ui.lvclass">)
        n147 = call "picture.clear.vi"("Keep Keyboard? (T)"=FALSE, "error in"=w428, "midi-ui in"=w426) -> ("error out"=w429:errorcluster, "midi-ui out"=w430:refnum<class "midi-ui.lvclass">)  [unwired: 7 in]
        n148 = call "picture.publish.vi"("error in"=w429, "midi-ui in"=w430) -> ("error out"=w427:errorcluster, "midi-ui out"=w423:refnum<class "midi-ui.lvclass">)  [unwired: 8 in]
        n149 = Bundle By Name(cluster=w425, "MIDI UI"=w423) -> (w424:T3)
        n150 = call <vilib>:"Add State(s) to Queue__jki_lib_state_machine.vi"("State(s) in (\"\")"=w433) -> ("States Out"=w432:string)  [unwired: 14 in]
      }
      frame "MIDI UI: Keyboard Note On" {
        n151 = disable-structure shown="Enabled" {
          disable-tunnel: w439 -> [w451 w452]
          disable-tunnel: [w450 w452] -> w438
          disable-tunnel: w436 -> [w447 _]
          disable-tunnel: [w446 _] -> w435
          disable-tunnel: w434 -> [w443 _]
          frame Disabled {
            n152 = Search and Replace String(input string=w443, search string="~", replace string="#" ("replace string (\"\")")) -> (result string=w442:string)  [unwired: 5 in, 3 out]
            n153 = Unbundle By Name(w451) -> ("MIDI UI"=w449:refnum<class "midi-ui.lvclass">)
            n154 = call "keyboard.NoteOn.vi"("error in (no error)"=w447, "Note Value"=w442, "midi-ui in"=w449) -> ("error out"=w446:errorcluster, "midi-ui out"=w448:refnum<class "midi-ui.lvclass">)  [unwired: 7 in]
            n155 = Bundle By Name(cluster=w451, "MIDI UI"=w448) -> (w450:T3)
          }
          frame Enabled {
          }
        }
        n156 = call <vilib>:"Add State(s) to Queue__jki_lib_state_machine.vi"("State(s) in (\"\")"=w441) -> ("States Out"=w440:string)  [unwired: 14 in]
      }
      frame "MIDI UI: Music Note On" {
        n157 = disable-structure shown="Disabled" {
          disable-tunnel: w458 -> [w467 w468]
          disable-tunnel: [w466 w468] -> w457
          disable-tunnel: w455 -> [w463 _]
          disable-tunnel: [w462 _] -> w454
          disable-tunnel: w453 -> [w461 _]
          frame Disabled {
            n158 = Unbundle By Name(w467) -> ("MIDI UI"=w465:refnum<class "midi-ui.lvclass">)
            n159 = call "music.NoteOn.vi"("error in (no error)"=w463, "uid"=w461, "midi-ui in"=w465) -> ("error out"=w462:errorcluster, "midi-ui out"=w464:refnum<class "midi-ui.lvclass">)  [unwired: 7 in]
            n160 = Bundle By Name(cluster=w467, "MIDI UI"=w464) -> (w466:T3)
          }
          frame Enabled {
          }
        }
        n161 = call <vilib>:"Add State(s) to Queue__jki_lib_state_machine.vi"("State(s) in (\"\")"=w460) -> ("States Out"=w459:string)  [unwired: 14 in]
      }
      frame "MIDI UI: Keyboard Note Off" {
        n162 = disable-structure shown="Enabled" {
          disable-tunnel: w474 -> [w486 w487]
          disable-tunnel: [w485 w487] -> w473
          disable-tunnel: w471 -> [w482 _]
          disable-tunnel: [w481 _] -> w470
          disable-tunnel: w469 -> [w478 _]
          frame Disabled {
            n163 = Search and Replace String(input string=w478, search string="~", replace string="#" ("replace string (\"\")")) -> (result string=w477:string)  [unwired: 5 in, 3 out]
            n164 = Unbundle By Name(w486) -> ("MIDI UI"=w484:refnum<class "midi-ui.lvclass">)
            n165 = call "keyboard.NoteOff.vi"("error in (no error)"=w482, "piano note"=w477, "midi-ui in"=w484) -> ("error out"=w481:errorcluster, "midi-ui out"=w483:refnum<class "midi-ui.lvclass">)  [unwired: 7 in]
            n166 = Bundle By Name(cluster=w486, "MIDI UI"=w483) -> (w485:T3)
          }
          frame Enabled {
          }
        }
        n167 = call <vilib>:"Add State(s) to Queue__jki_lib_state_machine.vi"("State(s) in (\"\")"=w476) -> ("States Out"=w475:string)  [unwired: 14 in]
      }
      frame "MIDI UI: Music Note Off" {
        n168 = disable-structure shown="Enabled" {
          disable-tunnel: w493 -> [w502 w503]
          disable-tunnel: [w501 w503] -> w492
          disable-tunnel: w490 -> [w498 _]
          disable-tunnel: w489 -> [w497 _]
          disable-tunnel: [w496 _] -> w488
          frame Disabled {
            n169 = Unbundle By Name(w502) -> ("MIDI UI"=w500:refnum<class "midi-ui.lvclass">)
            n170 = call "music.NoteOff.vi"("error in (no error)"=w497, "uid"=w498, "midi-ui in"=w500) -> ("error out"=w496:errorcluster, "midi-ui out"=w499:refnum<class "midi-ui.lvclass">)  [unwired: 7 in]
            n171 = Bundle By Name(cluster=w502, "MIDI UI"=w499) -> (w501:T3)
          }
          frame Enabled {
          }
        }
        n172 = call <vilib>:"Add State(s) to Queue__jki_lib_state_machine.vi"("State(s) in (\"\")"=w495) -> ("States Out"=w494:string)  [unwired: 14 in]
      }
      frame "---------- MIDI FILE ----------" {
        n173 = call <vilib>:"Add State(s) to Queue__jki_lib_state_machine.vi"("State(s) in (\"\")"=w506) -> ("States Out"=w507:string)  [unwired: 14 in]
      }
      frame "MIDI FILE: Open File" {
        n174 = call "file.open.vi"("error in"=w516) -> ("error out"=w513:errorcluster, "Path to MIDI File"=w510:path, "midi-file out"=w512:refnum<class "midi-file.lvclass">)  [unwired: 8 in]
        n175 = Strip Path(path=w510) -> (name=→"File Name":string)  [unwired: 1 out]
        n176 = Bundle By Name(cluster=w515, "MIDI FILE"=w512) -> (w514:T3)
        n177 = call <vilib>:"Add State(s) to Queue__jki_lib_state_machine.vi"("State(s) in (\"\")"=w517) -> ("States Out"=w518:string)  [unwired: 14 in]
      }
      frame "MIDI FILE: Analyse File" {
        n178 = Unbundle By Name(w526) -> ("MIDI FILE"=w525:refnum<class "midi-file.lvclass">, "midi-file-events"=w519:refnum<class "midi-file-events.lvclass">)
        n179 = call "track_chunk.read.vi"("error in"=w524, "midi-file-events in"=w519, "midi-file in"=w525) -> ("error out"=w523:errorcluster, "midi-file-events out"=w520:refnum<class "midi-file-events.lvclass">, "midi-file out"=w522:refnum<class "midi-file.lvclass">)  [unwired: 6 in]
        n180 = Bundle By Name(cluster=w526, "MIDI FILE"=w522, "midi-file-events"=w520) -> (w527:T3)
        n181 = call <vilib>:"Add State(s) to Queue__jki_lib_state_machine.vi"("State(s) in (\"\")"=w528) -> ("States Out"=w529:string)  [unwired: 14 in]
      }
      frame "MIDI FILE: Close File" {
        n182 = Unbundle By Name(w534) -> ("MIDI FILE"=w533:refnum<class "midi-file.lvclass">)
        n183 = call "file.close.vi"("error in"=w532, "midi-file in"=w533) -> ("error out"=w531:errorcluster)  [unwired: 9 in]
        n184 = call <vilib>:"Add State(s) to Queue__jki_lib_state_machine.vi"("State(s) in (\"\")"=w535) -> ("States Out"=w536:string)  [unwired: 14 in]
      }
      frame "---------- MIDI OUT ----------" {
        n185 = call <vilib>:"Add State(s) to Queue__jki_lib_state_machine.vi"("State(s) in (\"\")"=w540) -> ("States Out"=w541:string)  [unwired: 14 in]
      }
      frame "MIDI OUT: Connect" {
        n186 = Unbundle By Name(w547) -> ("MIDI"=w549:refnum<class "midi.lvclass">)
        n187 = call "midiOutOpen.vi"("error in"=w550, "DeviceID"="Midi Device", "midi in"=w549) -> ("error out"=w544:errorcluster, "midi out"=w546:refnum<class "midi.lvclass">)  [unwired: 7 in]
        n188 = Not(x=w544) -> (.not. x?=w543:bool)
        "Connected?" <- w543
        n189 = Bundle By Name(cluster=w547, "MIDI"=w546, "midi connected?"=w543) -> (w548:T3)
        n190 = call <vilib>:"Add State(s) to Queue__jki_lib_state_machine.vi"("State(s) in (\"\")"=w551) -> ("States Out"=w552:string)  [unwired: 14 in]
      }
      frame "MIDI OUT: Disconnect" {
        w553 = FALSE ("midi connected?")
        n191 = Unbundle By Name(w557) -> ("MIDI"=w558:refnum<class "midi.lvclass">)
        n192 = call "midiOutClose.vi"("error in"=w556, "midi in"=w558) -> ("error out"=w555:errorcluster, "midi out"=w559:refnum<class "midi.lvclass">)  [unwired: 8 in]
        n193 = Bundle By Name(cluster=w557, "midi connected?"=w553, "MIDI"=w559) -> (w560:T3)
        n194 = local write "Connected?"(w553) -> ()
        n195 = call <vilib>:"Add State(s) to Queue__jki_lib_state_machine.vi"("State(s) in (\"\")"=w561) -> ("States Out"=w562:string)  [unwired: 14 in]
      }
      frame "---------- MIDI Player ----------" {
        n196 = call <vilib>:"Add State(s) to Queue__jki_lib_state_machine.vi"("State(s) in (\"\")"=w566) -> ("States Out"=w567:string)  [unwired: 14 in]
      }
      frame "MIDI OUT: Launch Player" {
        n197 = Unbundle By Name(w577) -> ("midiPlayer"=w574:refnum<class "midiPlayer.lvclass">, "MIDI"=w573:refnum<class "midi.lvclass">, "MIDI UI"=w572:refnum<class "midi-ui.lvclass">, "midi-file-events"=w570:refnum<class "midi-file-events.lvclass">)
        n198 = property class="midiPlayer.lvclass"(reference=w574, error in=w568, "midi"=w573, "midi-ui"=w572, "midi-file-events"=w570) -> (reference out=w571:refnum<class "midiPlayer.lvclass">, error out=w569:errorcluster)
        n199 = call "midiOutPlayer.Launch.vi"("error in"=w569, "midiPlayer in"=w571) -> ("error out"=w578:errorcluster, "midiPlayer out"=w575:refnum<class "midiPlayer.lvclass">)  [unwired: 8 in]
        n200 = Bundle By Name(cluster=w577, "midiPlayer"=w575) -> (w576:T3)
        n201 = call <vilib>:"Add State(s) to Queue__jki_lib_state_machine.vi"("State(s) in (\"\")"=w580) -> ("States Out"=w581:string)  [unwired: 14 in]
      }
      frame "MIDI OUT: Play" {
        n202 = Unbundle By Name(w587) -> ("midiPlayer"=w583:refnum<class "midiPlayer.lvclass">)
        n203 = call "midiOutPlayer.msg.Play.vi"("error in (no error)"=w586, "midiPlayer in"=w583) -> ("error out"=w585:errorcluster, "midiPlayer out"=w582:refnum<class "midiPlayer.lvclass">)  [unwired: 8 in]
        n204 = Bundle By Name(cluster=w587, "midiPlayer"=w582) -> (w584:T3)
        n205 = call <vilib>:"Add State(s) to Queue__jki_lib_state_machine.vi"("State(s) in (\"\")"=w589) -> ("States Out"=w590:string)  [unwired: 14 in]
      }
    }
  }
